vi "Config Global.vi"() -> ()   [LabVIEW 2015, in "Configuration Tool.lvlib"]
uses:
  Configuration Tool.lvlib
panel:
  in  "VS Version":string="2015"
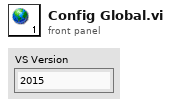
[diagram p1: front panel]
diagram:
